vi "FindLastWednesday.vi"(1 "current time":timestamp) -> (0 "Most Recent Wednesday":timestamp)   [LabVIEW 2022 SP3]
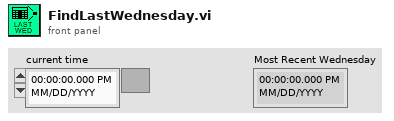
[diagram p1: front panel]
types:
  T1 = typedef "LVDateTimeRec.ctl" = cluster{"fractional second":dbl, "second":i32, "minute":i32, "hour":i32, "day of month":i32, "month":i32, "year":i32, "day of week":i32, "day of year":i32, "DST":i32}
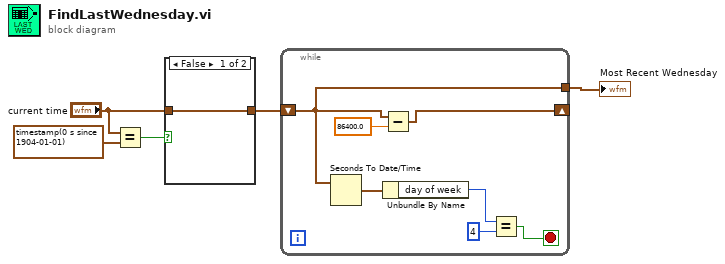
[diagram p0: block diagram]
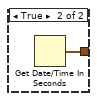
[diagram p2: hidden frame]
diagram:
  n1 = Equal?(x="current time", y=timestamp(0 s since 1904-01-01)) -> (x = y?=w2:bool)
  n2 = case shown="False" w2 {
    tunnel: [w6 w7] -> w5
    tunnel: "current time" -> [w6 _]
    frame False {
    }
    frame True {
      n3 = Get Date/Time In Seconds() -> (seconds since 1Jan1904=w7:timestamp)
    }
  }
  n4 = while {
    shift-right: [w9] -> _
    shift-left: w5 -> [w8]
    tunnel: [w8] -> w4
    stop <- w12 stop-if-true
    n5 = Seconds To Date/Time(time stamp (now)=w8) -> (date time rec=w14:T1)  [unwired: 1 in]
    n6 = Subtract(x=w8, y=86400.0) -> (x-y=w9:timestamp)
    n7 = Unbundle By Name(w14) -> ("day of week"=w13:i32)
    n8 = Equal?(x=w13, y=4) -> (x = y?=w12:bool)
  }
  "Most Recent Wednesday" <- w4
